vi "PF_1.vi"() -> ()   [LabVIEW 2020]
uses:
  Control 1.ctl
  <vilib>/Instr/_visa.llb/VISA Configure Serial Port (Instr).vi
panel:
  in  "Selección Puerto":refnum<visa-resource-name>
  out "Temperatura actual":dbl format="%#_13g"
  out "Temperatura":dbl(graph)
  out "Voltaje":i32(graph)
  out "?":string="Histerisis"
  in  "?":bool
  in  "Temperatura Mínima":dbl
  in  "Temperatura Máxima":dbl
  out "Usuario confirmado":string
  out "Acceso permitido":bool
  in  "Tabla de usuarios":T1
  in  "Contraseña":string
  in  "Usuario":string
  # "Proyecto Final - Instrumentación Virtual Aplicada\n\"Controlador de temperatura con histéresis configurable por medio de interfaz gráfica\""
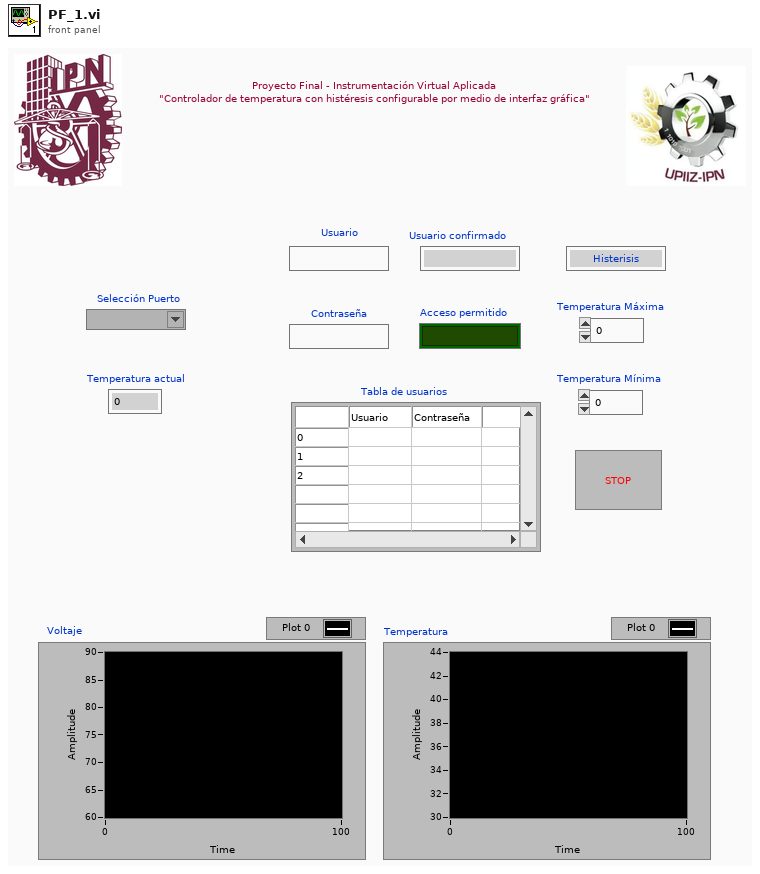
[diagram p1: front panel]
types:
  T1 = typedef "Control 1.ctl" = string[][]
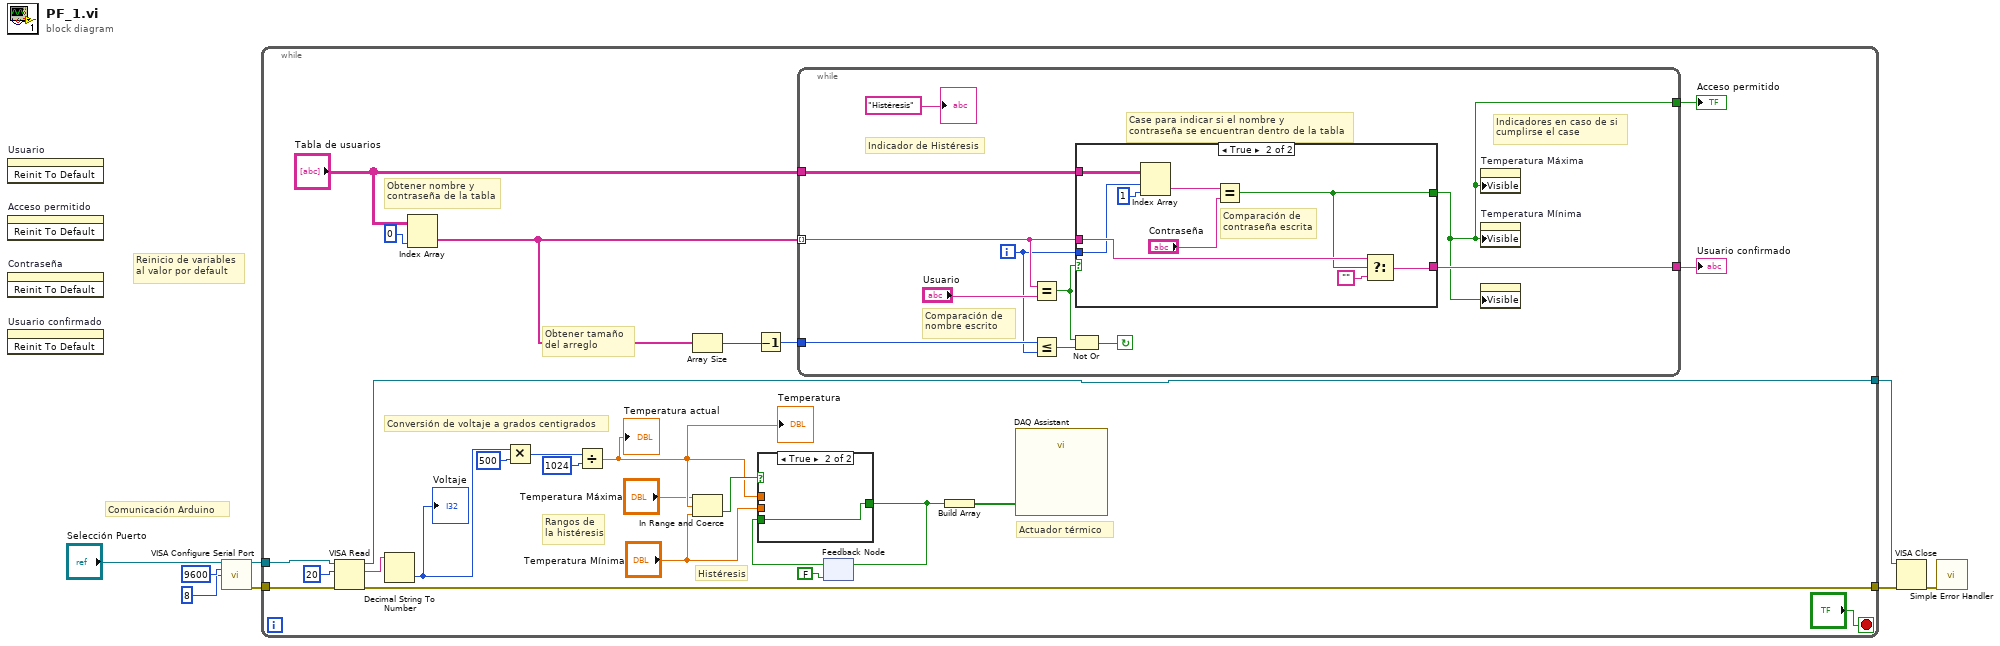
[diagram p0: block diagram]
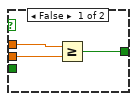
[diagram p2: hidden frame]
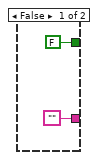
[diagram p3: hidden frame]
diagram:
  # "Reinicio de variables \nal valor por default"
  # "Comunicación Arduino"
  n1 = invoke on="Usuario" class="Str" method="Reinit To Default"() -> ()  [unwired: 3 in, 3 out]
  n2 = invoke on="Acceso permitido" class="Bool (strict)" method="Reinit To Default"() -> ()  [unwired: 3 in, 3 out]
  n3 = invoke on="Contraseña" class="Str" method="Reinit To Default"() -> ()  [unwired: 3 in, 3 out]
  n4 = invoke on="Usuario confirmado" class="Str" method="Reinit To Default"() -> ()  [unwired: 3 in, 3 out]
  n5 = call-poly "VISA Configure Serial Port"("VISA resource name"="Selección Puerto", "baud rate (9600)"=u32 9600, "data bits (8)"=u16 8) -> ("VISA resource name out"=w5:refnum<visa-resource-name>, "error out"=w4:errorcluster)  [unwired: 11 in]
  n6 = while {
    tunnel: w5 -> [w17]
    tunnel: w4 -> [w16]
    tunnel: [w9] -> w2
    tunnel: [w10] -> w1
    stop <- "?" stop-if-true
    # "Actuador térmico"
    # "Rangos de\nla histéresis"
    # "Histéresis"
    # "Conversión de voltaje a grados centigrados"
    # "Obtener tamaño \ndel arreglo"
    # "Obtener nombre y \ncontraseña de la tabla"
    n7 = VISA Read(VISA resource name=w17, byte count=u32 20, error in (no error)=w16) -> (VISA resource name out=w9:refnum<visa-resource-name>, read buffer=w25:string, error out=w10:errorcluster)  [unwired: 1 out]
    n8 = Decimal String To Number(string=w25) -> (number=w24:i32)  [unwired: 2 in, 1 out]
    "Voltaje" <- w24
    n9 = Index Array(array="Tabla de usuarios", index (col)=0 ("disabled index (col)")) -> (element=w32:string[])  [unwired: 1 in]
    n10 = Multiply(x=w24, y=500) -> (x*y=w22:i32)
    n11 = Divide(x=w22, y=1024) -> (x/y=w18:dbl)
    "Temperatura" <- w18
    "Temperatura actual" <- w18
    n12 = Array Size(array=w32) -> (size(s)=w34:i32)
    n13 = In Range and Coerce(upper limit="Temperatura Máxima", x=w18, lower limit="Temperatura Mínima") -> (In Range?=w19:bool)  [unwired: 1 out]
    n14 = Decrement(x=w34) -> (x-1=w33:i32)
    n15 = while {
      tunnel: w33 -> [w48]
      tunnel: w32 -> [w46] mode=indexing
      tunnel: [w39] -> w31
      tunnel: [w45] -> w30
      tunnel: "Tabla de usuarios" -> [w44]
      i -> [w43]
      stop <- w41 continue-if-true
      # "Indicador de Histéresis"
      # "Indicadores en caso de si \ncumplirse el case"
      # "Case para indicar si el nombre y \ncontraseña se encuentran dentro de la tabla"
      # "Comparación de \nnombre escrito"
      n16 = Equal?(x=w46, y="Usuario") -> (x = y?=w42:bool)
      n17 = Less Or Equal?(x=w48, y=w43) -> (x <= y?=w49:bool)
      n18 = Not Or(1:w49, 2:w42) -> (0:w41:bool)
      n19 = case shown="True" w42 {
        tunnel: w44 -> [_ w54]
        tunnel: w46 -> [_ w57]
        tunnel: [FALSE w56] -> w39
        tunnel: ["" w55] -> w45
        tunnel: w43 -> [_ w53]
        frame False {
        }
        frame True {
          # "Comparación de \ncontraseña escrita"
          n20 = Index Array(array=w54, index (row)=w53, index (col)=1) -> (element=w58:string)
          n21 = Equal?(x=w58, y="Contraseña") -> (x = y?=w56:bool)
          n22 = Select(t=w57, s=w56, f="") -> (s? t:f=w55:string)
        }
      }
      n23 = property on="Temperatura Máxima" class="DigNum (strict)"("Visible"=w39) -> ()  [unwired: 2 in, 2 out]
      n24 = property on="Temperatura Mínima" class="DigNum (strict)"("Visible"=w39) -> ()  [unwired: 2 in, 2 out]
      n25 = property class="Str"("Visible"=w39) -> ()  [unwired: 2 in, 2 out]
      "?" <- "Histéresis"
    }
    "Acceso permitido" <- w31
    "Usuario confirmado" <- w30
    n26 = feedback #1(FALSE) -> (w20:bool)
    n27 = case shown="True" w19 {
      tunnel: w18 -> [w37 _]
      tunnel: "Temperatura Mínima" -> [w36 _]
      tunnel: [w35 w38] -> w11
      tunnel: w20 -> [_ w38]
      frame False {
        n28 = Greater Or Equal?(x=w37, y=w36) -> (x >= y?=w35:bool)
      }
      frame True {
      }
    }
    n29 = feedback-in #1(w11) -> ()
    n30 = Build Array(w11) -> (w12:bool[])
    n31 = call "DAQ Assistant"("data"=w12) -> ()  [unwired: 17 in, 2 out]
  }
  n32 = VISA Close(VISA resource name=w2, error in (no error)=w1) -> (error out=w3:errorcluster)
  n33 = call <vilib>:"Simple Error Handler.vi"("error in (no error)"=w3) -> ()  [unwired: 4 in, 5 out]
